vi "CFU_7_Potluri.vi"() -> ()   [LabVIEW 2016]
panel:
  out "Numeric 2":i32
  in  "Numeric":i32
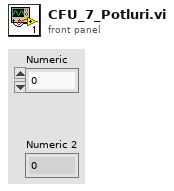
[diagram p1: front panel]
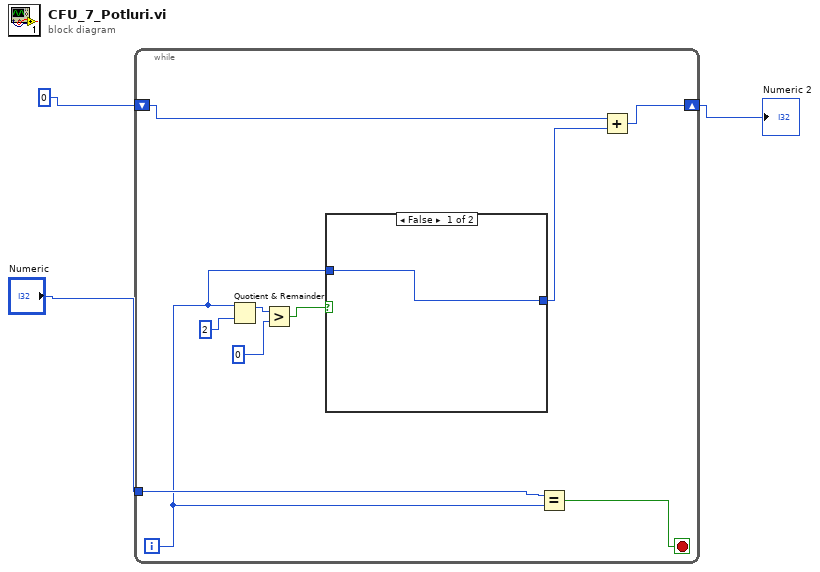
[diagram p0: block diagram]
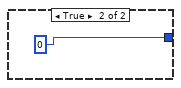
[diagram p2: hidden frame]
diagram:
  n1 = while {
    shift-right: [w7] -> w1
    shift-left: 0 -> [w8]
    tunnel: "Numeric" -> [w6]
    i -> [w5]
    stop <- w4 stop-if-true
    n2 = Quotient & Remainder(x=w5, y=2) -> (x-y*floor(x/y)=w12:i32)  [unwired: 1 out]
    n3 = Greater?(x=w12, y=0) -> (0:w10:bool)
    n4 = case shown="False" w10 {
      tunnel: w5 -> [w14 _]
      tunnel: [w14 0] -> w9
      frame False {
      }
      frame True {
      }
    }
    n5 = Equal?(x=w6, y=w5) -> (x = y?=w4:bool)
    n6 = Add(x=w8, y=w9) -> (x+y=w7:i32)
  }
  "Numeric 2" <- w1
